vi "Main-e.vi"() -> ()   [LabVIEW 2015]
doc: "This template is for the Queued Message Handler design pattern.\n\nThe Event Handling Loop generates messages based on user interface actions.\n\nThe Message Handling Loop processes messages generated by the Event Handling Loop, or by other messages. The messages are string values, so new messages can be added easily to the Message Cases case structure in the Message Handling Loop. Each message cluster can also provide an optional value for Message Data, which is a variant that can be converted to whatever message-specific data is required."
uses:
  controls/UI Data.ctl
  <vilib>/Platform/TimedLoop/XDataNode/timing_clust.ctl
  <vilib>/Platform/TimedLoop/XDataNode/nitl_modes.ctl
  <vilib>/Platform/TimedLoop/XDataNode/wakeup.ctl
  support/Message Queue/Enqueue Message (Single).vi
  <vilib>/Utility/error.llb/Error Cluster From Error Code.vi
  <vilib>/ErrorRing/Error Ring.xnode
  <vilib>/platform/TimedLoop/XDataNode/XDataNode.xnode
  support/Message Queue/Message Queue.lvlib
  support/User Events/User Events.lvlib
  <userlib>/cameraLibrary/cameraLibrary.lvlib
  <vilib>/Platform/TimedLoop/XDataNode/XDNodeRunTimeDep.lvlib
panel:
  out "status out":u32
  in  "Stop Button":bool
  out "Array Temp":i32
  in  "Set Temp":i32
  out "Image":T1(plugin-control)
  out "loopClosed?":bool
  out "ROIUpdated?":bool
  in  "closeLoopButton":bool
  in  "Subframe":dbl(ring) items=["Slow"=0.01, "Medium"=0.005, "Fast"=0.001]
  in  "Full frame":dbl
  out "Y Fiber Position":i32
  out "X Fiber Pos.":i32
  in  "Y Dimension":i16
  in  "X Dimension":i16
  in  "roiButton":bool
  in  "fullFrameButton":bool
  out "Display":string
  in  "abortButton":bool
  in  "subFrameButton":bool
  in  "Exit":bool
  # "Status indicators"
  # "Loop Closed"
  # "ROI Up-to-date"
  # "Timing parameters"
  # "ROI parameters"
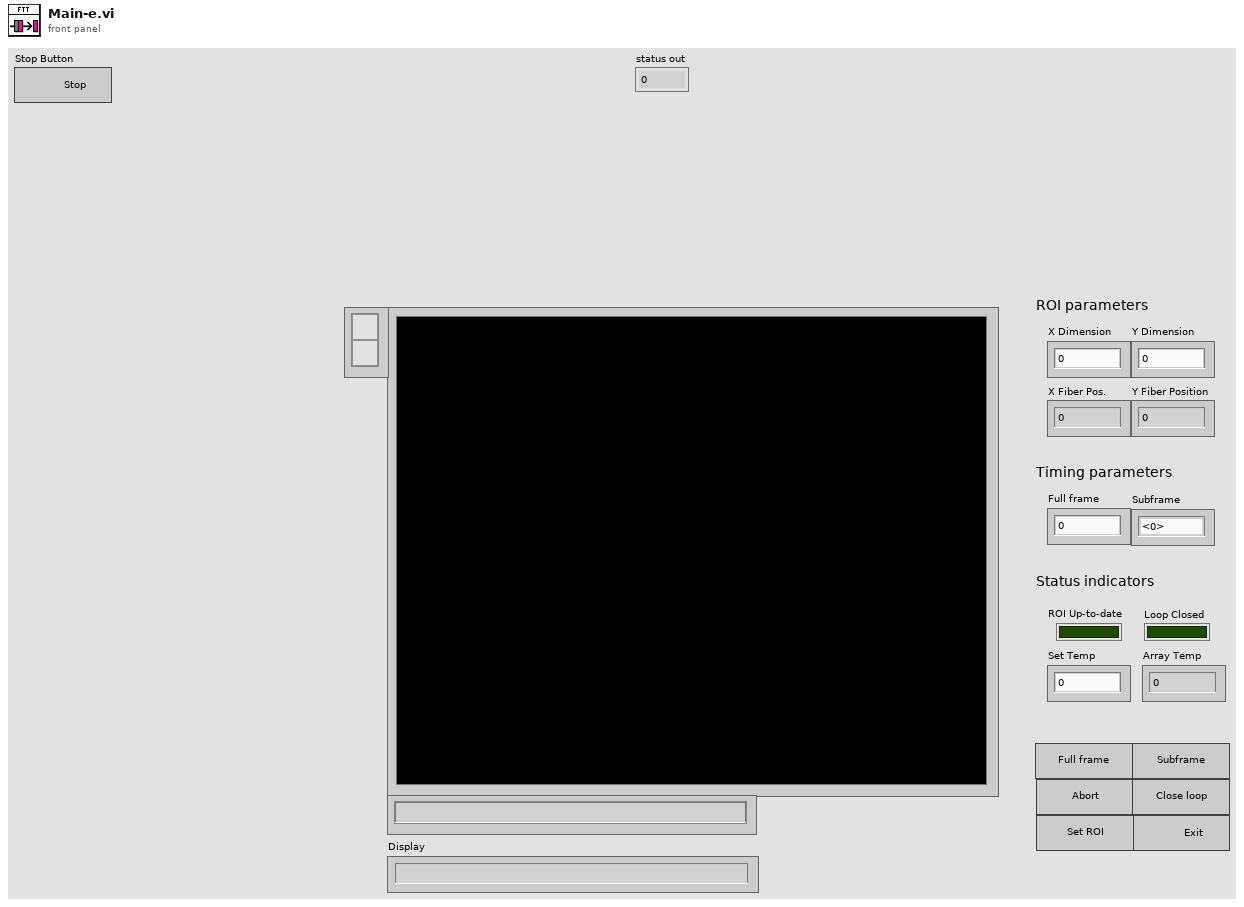
[diagram p1: front panel]
types:
  T1 = typedef "IMAQ Image.ctl" = refnum<image>
  T2 = typedef "Image Type" = u32
  T3 = typedef "UI Data.ctl" = cluster{"full Frame Button Ref":refnum<vi>, "subFrame Button Ref":refnum<vi>, "closed Loop Button Ref":refnum<vi>, "ROI button Ref":refnum<vi>, "abort Button Ref":refnum<vi>, "exit Button Ref":refnum<vi>, "acquiring":bool, " acquiring Ref":refnum<vi>, " ROI Updated Ref":refnum<vi>, "loop Closed Ref":refnum<vi>, "ROI":cluster{"X dimension":i16, "Y dimension":i16, "X binning":i16, "Y binning":i16, "X start":i16, "Y start":i16}, "String <Replace Me>":string, "Data Display Ref":refnum<vi>, "Image Ref":refnum<vi>}
  T4 = typedef "UI Events.ctl" = cluster{"User Event - Stop":refnum<user-event>, "User Event - Abort":refnum<user-event>, "User Event - UpdateTemp":refnum<user-event>}
  T5 = typedef "Message Queue.lvlib/All Message Queues.ctl" = cluster{"UI":refnum<queue>, "DataDisplay":refnum<queue>}
  T6 = typedef "XDNodeRunTimeDep.lvlib/timing_clust.ctl" = cluster{"Expected End [f-1]":u64, "Actual End [f-1]":u64, "Finished Late? [f-1]":bool, "Expected End [i-1]":u64, "Actual End [i-1]":u64, "Finished Late? [i-1]":bool, "Expected Start [i]":u64, "Actual Start [i]":u64, "Expected Start [f]":u64, "Actual Start [f]":u64, "Source Name":string, "Structure Name":string, "Period":i64, "Deadline":i64, "Offset":i64, "Start":i64, "Priority":i32, "Timeout":i32, "Mode":T7, "Wakeup Reason":T8, "Error":errorcluster, "Source Type":string, "Secondary Source Type":string, "Global End Time":u64, "Global Start Time":u64, "Frame Duration":u64, "Iteration Duration":u64, "Assigned CPU":i32, "I/O Scan Engine Mode":u32}
  T7 = typedef "XDNodeRunTimeDep.lvlib/nitl_modes.ctl" = enum32{"No Change", "Process missed periods, maintain original phase", "Discard missed periods, maintain original phase", "Process missed periods, ignore original phase", "Discard missed periods, ignore original phase"}
  T8 = typedef "XDNodeRunTimeDep.lvlib/wakeup.ctl" = enum32{"Normal", "Aborted", "Asynchronous wakeup", "Timing source error", "Timed loop error", "Timeout"}
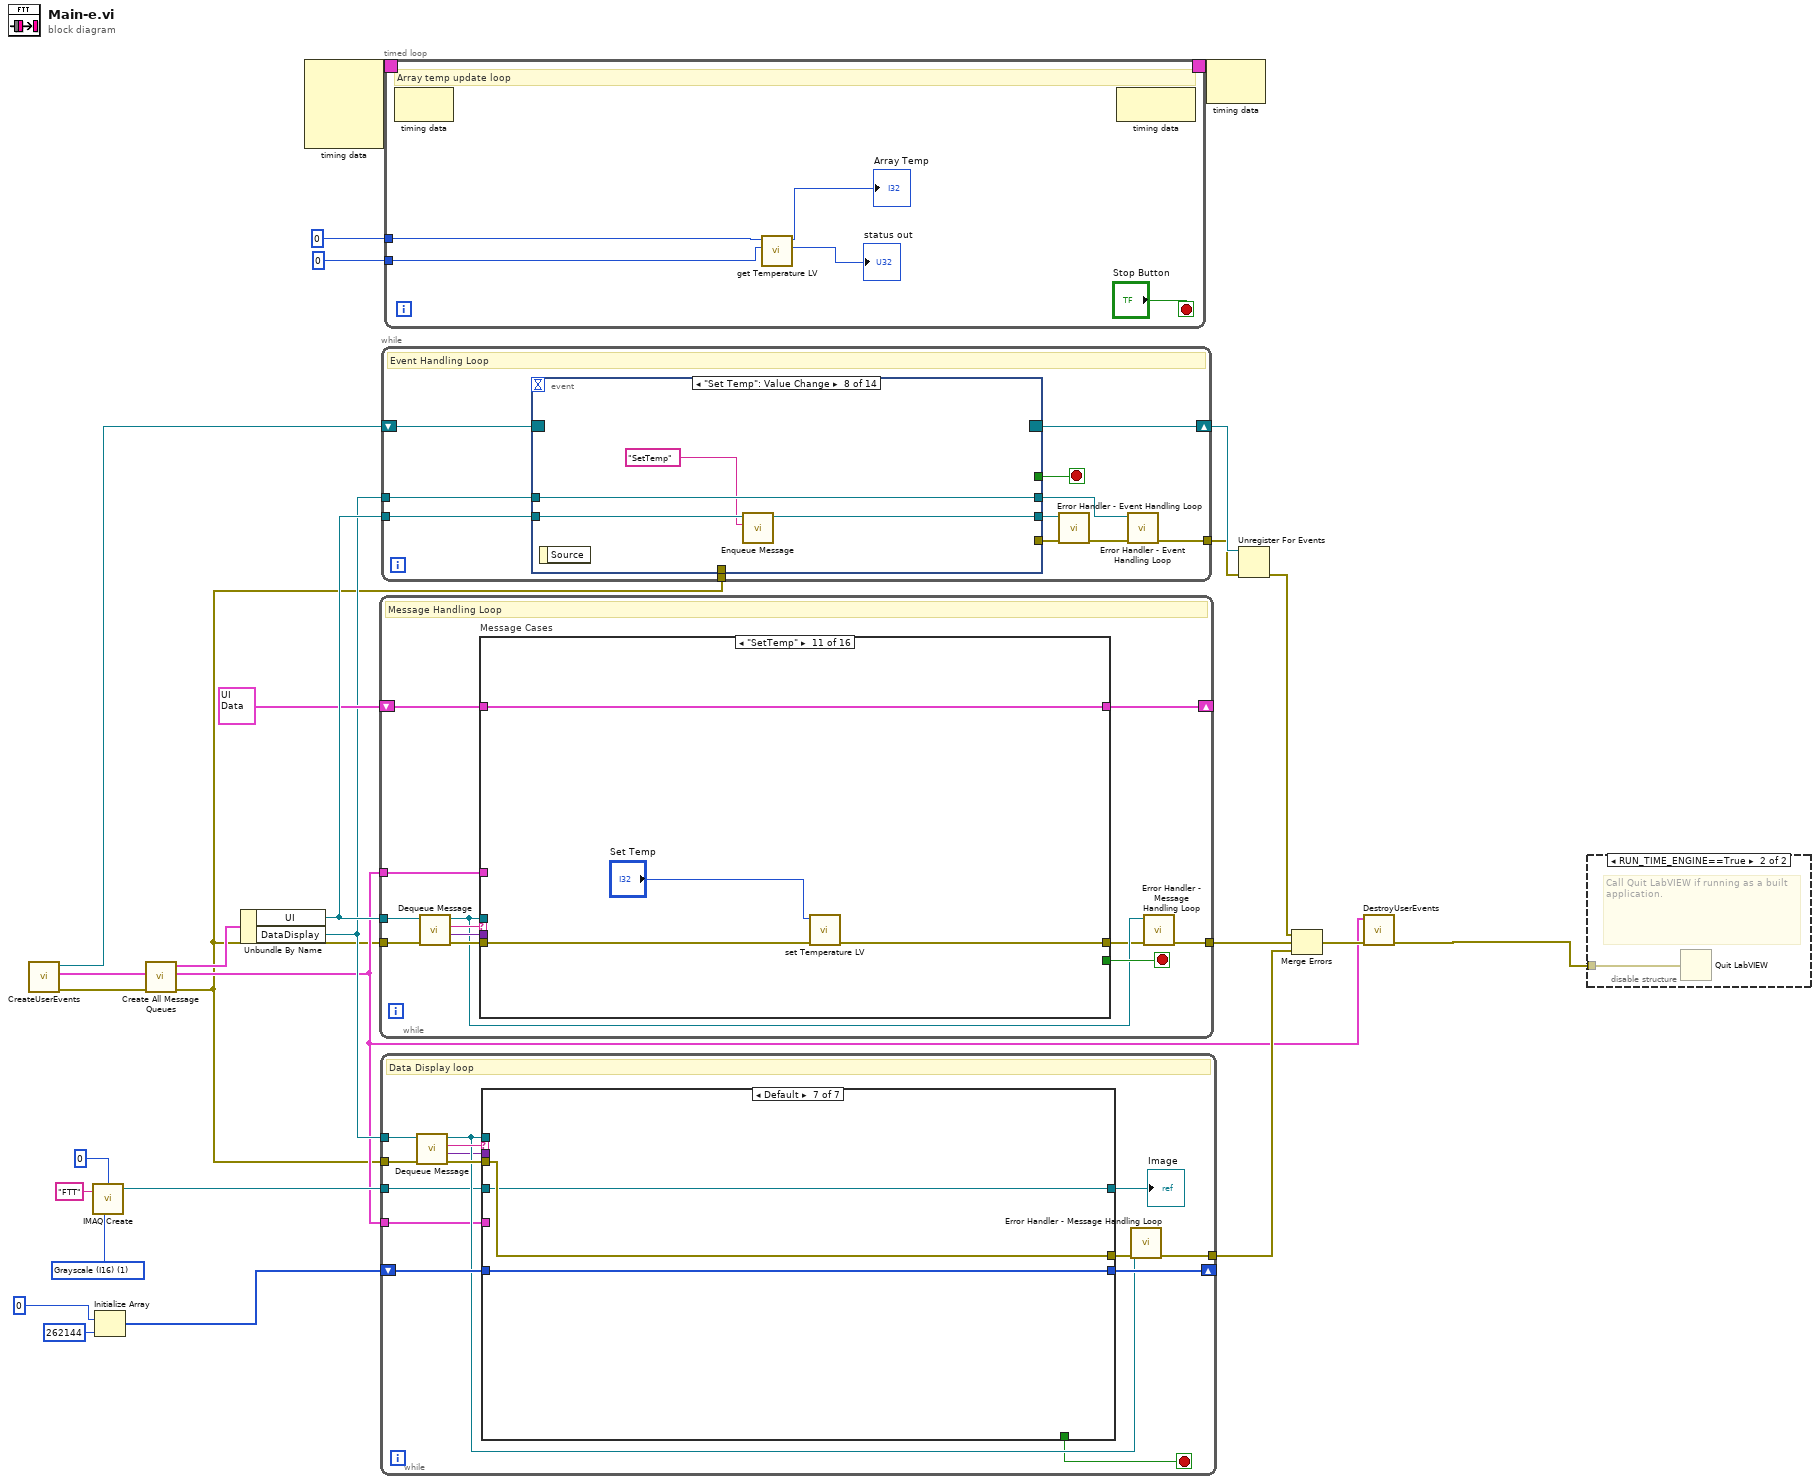
[diagram p0: block diagram]
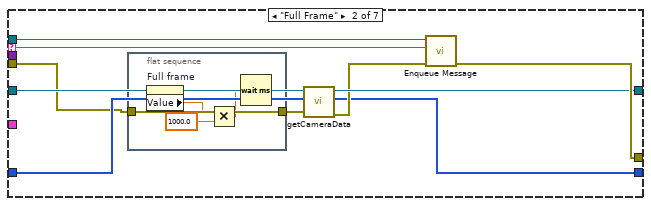
[diagram p3: hidden frame]
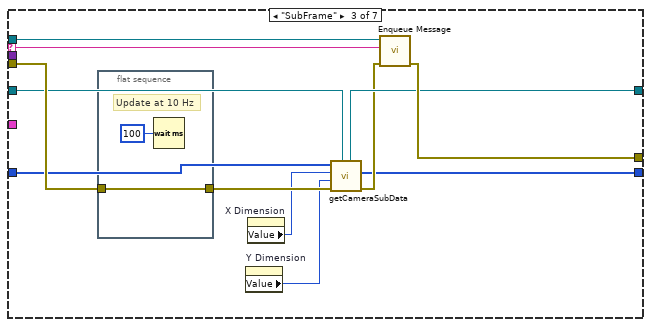
[diagram p4: hidden frame]
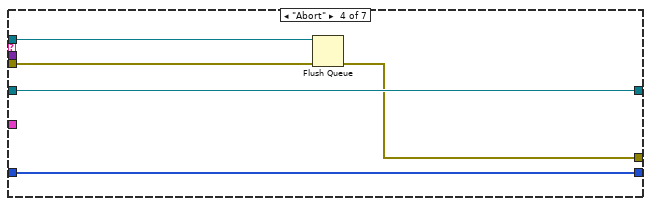
[diagram p5: hidden frame]
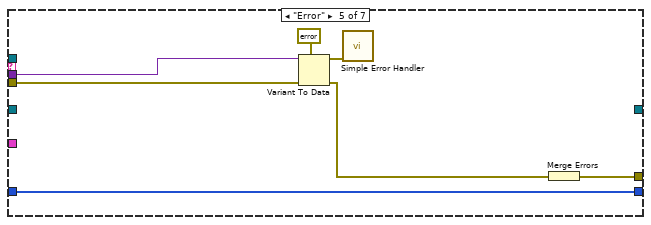
[diagram p6: hidden frame]
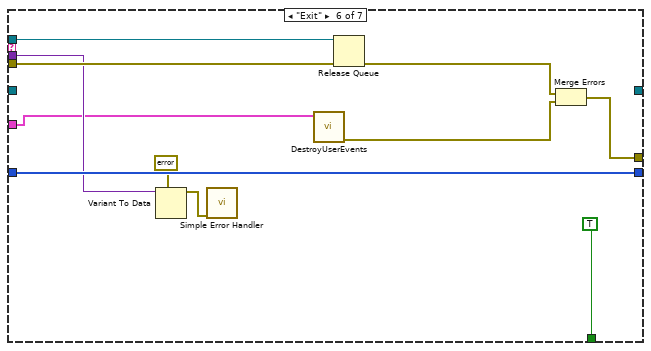
[diagram p7: hidden frame]
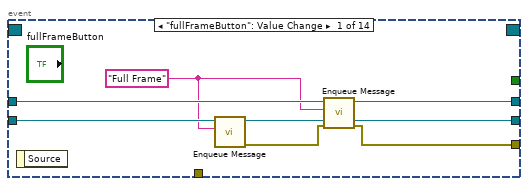
[diagram p9: hidden frame]
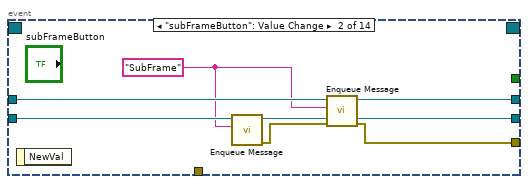
[diagram p10: hidden frame]
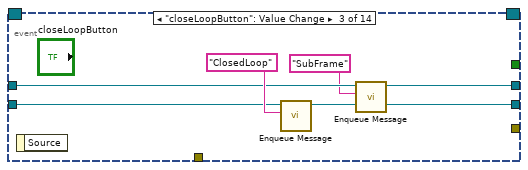
[diagram p11: hidden frame]
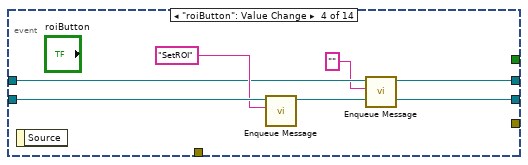
[diagram p12: hidden frame]
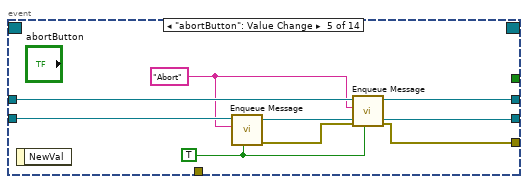
[diagram p13: hidden frame]
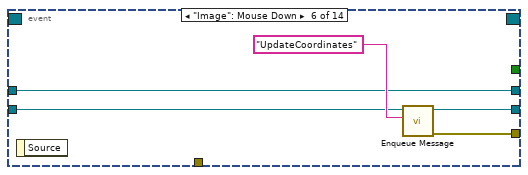
[diagram p14: hidden frame]
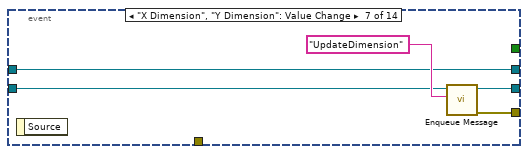
[diagram p15: hidden frame]
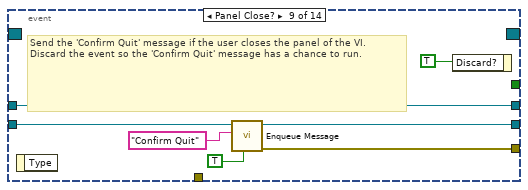
[diagram p16: hidden frame]
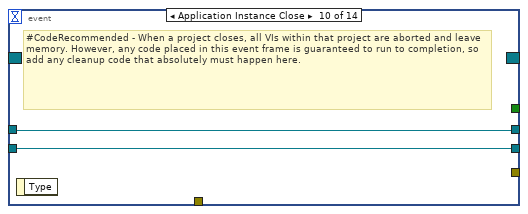
[diagram p17: hidden frame]
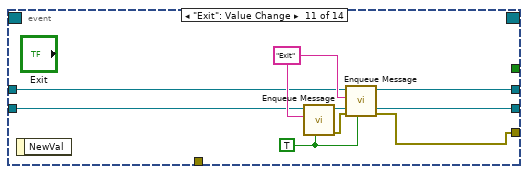
[diagram p18: hidden frame]
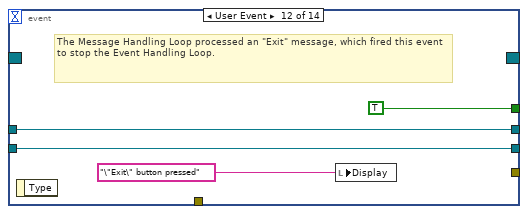
[diagram p19: hidden frame]
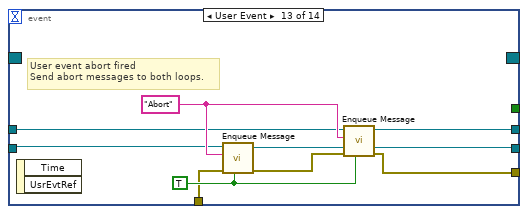
[diagram p20: hidden frame]
diagram:
  w13 = T2 1 items=["Grayscale (U8)", "Grayscale (I16)", "Grayscale (SGL)", "Complex (CSG)", "RGB (U32)", "HSL (U32)", "RGB (U64)", "Grayscale (U16)"] ("Image Type")
  n1 = call "CreateUserEvents.vi"() -> ("error out"=w23:errorcluster, "Event Cluster"=w7:T4, "Event Registration Refnum out"=w19:refnum<event-registration>)  [unwired: 9 in]
  n2 = call "IMAQ Create"("Border Size"=0, "Image Name"="FTT", "Image Type"=w13) -> ("New Image"=w10:T1)  [unwired: 2 in, 1 out]
  n3 = Initialize Array(u32 0, 262144 ("dimension size")) -> (w12:u32[])
  n4 = call "Create All Message Queues.vi"("error in (no error)"=w23) -> ("error out"=w5:errorcluster, "Message Queues out"=w26:T5)  [unwired: 9 in]
  n5 = Unbundle By Name(w26) -> ("UI"=w24:refnum<queue>, "DataDisplay"=w9:refnum<queue>)
  n6 = node-c288() -> (w4:T6)  [unwired: 4 in]
  n7 = while {
    tunnel: w24 -> [w33]
    shift-right: [w28] -> _
    shift-left: T3 {"full Frame Button Ref"=refnum, "subFrame Button Ref"=refnum, "closed Loop Button Ref"=refnum, "ROI button Ref"=refnum, "abort Button Ref"=refnum, "exit Button Ref"=refnum, "acquiring"=FALSE, " acquiring Ref"=refnum, " ROI Updated Ref"=refnum, "loop Closed Ref"=refnum, "ROI"={"X dimension"=0, "Y dimension"=0, "X binning"=0, "Y binning"=0, "X start"=0, "Y start"=0}, "String <Replace Me>"="", "Data Display Ref"=refnum, "Image Ref"=refnum} ("Data Cluster") -> [w38]
    tunnel: [w29] -> w25
    tunnel: w5 -> [w30]
    tunnel: w7 -> [w27]
    stop <- w37 stop-if-true
    # "Message Handling Loop"
    n8 = call "Dequeue Message.vi"("error in (no error)"=w30, "Message Queue"=w33) -> ("error out"=w36:errorcluster, "Message Data"=w34:variant, "Message"=w35:string, "dup Message Queue"=w32:refnum<queue>)  [unwired: 6 in]
    n9 = case "Message Cases" shown="\"SetTemp\"" w35 {
      selector: w35 -> [_ _ w71 _ _ _ _ _ _ _ _ _ _ _ _ w214]
      tunnel: w32 -> [w52 w66 w74 w90 _ _ _ _ _ _ _ _ w190 _ w213 _]
      tunnel: w36 -> [w51 w61 w73 w89 w108 w126 w142 w157 w159 w174 w179 w187 w194 w197 w204 _]
      tunnel: [w55 w67 w72 w93 w107 w125 w142 w157 w163 w175 w178 w181 w192 w195 w209 w215] -> w31
      tunnel: w38 -> [w54 w56 w76 w92 w110 w128 w140 w156 w161 w176 w180 w186 w193 w196 w212 w216]
      tunnel: [w45 w64 w70 w94 w109 w127 w139 w155 w162 w176 w180 w186 w193 w196 w212 w216] -> w28
      tunnel: [_ _ _ _ _ _ _ _ _ _ _ _ _ _ TRUE _] -> w37
      tunnel: w34 -> [_ _ _ _ _ _ _ _ _ w173 _ w185 _ _ w205 _]
      tunnel: w27 -> [_ _ w69 w88 w106 _ _ _ _ _ _ _ _ _ w200 _]
      frame "Initialize" {
        # "Initialize front panel buttons ."
        n10 = control-ref of="fullFrameButton"() -> (w50:refnum<vi>)
        n11 = control-ref of="subFrameButton"() -> (w49:refnum<vi>)
        n12 = control-ref of="closeLoopButton"() -> (w48:refnum<vi>)
        n13 = control-ref of="roiButton"() -> (w47:refnum<vi>)
        n14 = control-ref of="Display"() -> (w39:refnum<vi>)
        n15 = Bundle By Name(cluster=w54, "full Frame Button Ref"=w50, "subFrame Button Ref"=w49, "closed Loop Button Ref"=w48, "ROI button Ref"=w47, "Data Display Ref"=w39) -> (w46:T3)
        n16 = control-ref of="abortButton"() -> (w41:refnum<vi>)
        n17 = control-ref of="Exit"() -> (w42:refnum<vi>)
        n18 = control-ref of="ROIUpdated?"() -> (w40:refnum<vi>)
        n19 = control-ref of="loopClosed?"() -> (w43:refnum<vi>)
        n20 = control-ref of="Image"() -> (w44:refnum<vi>)
        n21 = Bundle By Name(cluster=w46, "abort Button Ref"=w41, "exit Button Ref"=w42, "ROI Updated Ref"=w40, "loop Closed Ref"=w43, "Image Ref"=w44) -> (w45:T3)
        n22 = call-poly "Enqueue Message.vi"("error in (no error)"=w51, "Message"="InitCamera", "Message Queue"=w52) -> ("error out"=w55:errorcluster)  [unwired: 7 in, 1 out]
      }
      frame "InitCamera" {
        w58 = 0.00125 items=["Slow"=0.01, "Medium"=0.035, "Fast"=0.00125] ("Subframe")
        w62 = i16 240 ("ROI.X start")
        w63 = i16 1 ("ROI.X binning")
        w59 = i16 32 ("ROI.X dimension")
        n23 = property on="Subframe" class="Ring (strict)"("Value"=w58) -> ()  [unwired: 2 in, 2 out]
        n24 = Bundle By Name(cluster=w56, "ROI.X dimension"=w59, "ROI.Y dimension"=w59, "ROI.X binning"=w63, "ROI.Y binning"=w63, "ROI.X start"=w62, "ROI.Y start"=w62) -> (w64:T3)
        n25 = call <userlib>:"initialize Camera LV.vi"("error in (no error)"=w61) -> ("error out"=w60:errorcluster)  [unwired: 10 in]
        n26 = property on="Full frame" class="DigNum (strict)"("Value"=0.5 ("Full frame")) -> ()  [unwired: 2 in, 2 out]
        n27 = property on="X Dimension" class="DigNum (strict)"("Value"=w59) -> ()  [unwired: 2 in, 2 out]
        n28 = property on="Y Dimension" class="DigNum (strict)"("Value"=w59) -> ()  [unwired: 2 in, 2 out]
        n29 = call-poly "Enqueue Message.vi"("error in (no error)"=w60, "Message Data"="Camera initialized" ("\"Do Something Else\" button pressed"), "Message"="Update Display", "Message Queue"=w66) -> ("error out"=w67:errorcluster)  [unwired: 6 in, 1 out]
      }
      frame "Full Frame" {
        n30 = Unbundle By Name(w76) -> ("acquiring"=w75:bool)
        n31 = case shown="True" w75 {
          tunnel: w76 -> [w81 w86]
          tunnel: [w81 w87] -> w70
          tunnel: w74 -> [_ _]
          tunnel: w73 -> [w78 w82]
          tunnel: [w77 w83] -> w72
          tunnel: w71 -> [_ _]
          tunnel: w69 -> [w80 _]
          frame True {
            # "Currently acquiring.\nFire user abort event."
            n32 = Unbundle By Name(w80) -> ("User Event - Abort"=w79:refnum<user-event>)
            n33 = call "Fire User Event - Abort.vi"("error in (no error)"=w78, "User Event - Abort"=w79) -> ("error out"=w77:errorcluster)  [unwired: 9 in]
          }
          frame False {
            # "Not currently acquiring.\nStart acquisition\nUpdate display parameters"
            n34 = call <userlib>:"acquire Full Frame LV.vi"("error in (no error)"=w82, "expTime"="Full frame") -> ("error out"=w84:errorcluster)  [unwired: 9 in]
            n35 = call "updateGUIDisplayParams.vi"("error in (no error)"=w84, "Data Cluster in"=w86) -> ("error out"=w83:errorcluster, "Data Cluster out"=w87:T3)  [unwired: 8 in]
          }
        }
      }
      frame "SubFrame" {
        # "Acquire a single frame from the camera"
        n36 = Unbundle By Name(w92) -> ("acquiring"=w91:bool)
        n37 = case shown="False" w91 {
          tunnel: w92 -> [w99 w100]
          tunnel: [w99 w103] -> w94
          tunnel: w90 -> [_ _]
          tunnel: w89 -> [w96 w105]
          tunnel: [w95 w101] -> w93
          tunnel: w88 -> [w98 _]
          frame True {
            # "Currently acquiring.\nFire user abort event.\nAborts current acquisition and stops data display loop"
            n38 = Unbundle By Name(w98) -> ("User Event - Abort"=w97:refnum<user-event>)
            n39 = call "Fire User Event - Abort.vi"("error in (no error)"=w96, "User Event - Abort"=w97) -> ("error out"=w95:errorcluster)  [unwired: 9 in]
          }
          frame False {
            n40 = call <userlib>:"acquire Sub Frame LV.vi"("error in (no error)"=w105, "expTime"="Subframe") -> ("error out"=w102:errorcluster)  [unwired: 9 in]
            n41 = call "updateGUIDisplayParams.vi"("error in (no error)"=w102, "Data Cluster in"=w100) -> ("error out"=w101:errorcluster, "Data Cluster out"=w103:T3)  [unwired: 8 in]
          }
        }
      }
      frame "ClosedLoop" {
        # "Handle closed loop button press. Start process FTT loop."
        n42 = Unbundle By Name(w110) -> ("acquiring"=w111:bool)
        n43 = case shown="True" w111 {
          tunnel: w110 -> [w116 w124]
          tunnel: [w113 w124] -> w109
          tunnel: w108 -> [w119 w121]
          tunnel: [w114 w120] -> w107
          tunnel: w106 -> [_ w123]
          frame False {
            # "Not acquiring, start closed\nloop acquisition"
            n44 = property on="Subframe" class="Ring (strict)"(error in=w119) -> (error out=w118:errorcluster, "Value"=w117:dbl)  [unwired: 1 in, 1 out]
            n45 = call <userlib>:"acquire Closed Loop LV.vi"("error in (no error)"=w118, "expTime"=w117) -> ("error out"=w115:errorcluster)  [unwired: 9 in]
            n46 = call "updateGUIDisplayParams.vi"("error in (no error)"=w115, "Data Cluster in"=w116) -> ("error out"=w114:errorcluster, "Data Cluster out"=w113:T3)  [unwired: 8 in]
            "loopClosed?" <- TRUE ("loopClosed?")
          }
          frame True {
            # "Currently acquiring.\nFire user abort event.\nAborts current acquisition and stops data display loop"
            n47 = Unbundle By Name(w123) -> ("User Event - Abort"=w122:refnum<user-event>)
            n48 = call "Fire User Event - Abort.vi"("error in (no error)"=w121, "User Event - Abort"=w122) -> ("error out"=w120:errorcluster)  [unwired: 9 in]
          }
        }
      }
      frame "SetROI" {
        # "Program camera with ROI values."
        n49 = Unbundle By Name(w128) -> ("acquiring"=w129:bool)
        n50 = case shown="True" w129 {
          tunnel: w128 -> [w131 w136]
          tunnel: [w131 w135] -> w127
          tunnel: w126 -> [w130 w134]
          tunnel: [w130 w133] -> w125
          frame True {
            # "Acquiring, do nothing\nShould be fixed with button masking"
          }
          frame False {
            # "Not acquiring, set ROI"
            n51 = call "setROI.vi"("error in (no error)"=w134, "FTTclusterIn"=w136) -> ("error out"=w133:errorcluster, "FTTclusterOut"=w135:T3)  [unwired: 8 in]
            "ROIUpdated?" <- TRUE ("ROIUpdated?")
          }
        }
      }
      frame "UpdateCoordinates" {
        # "Image clicked. If Acquiring, update coordinates.\nSignal ROI updated is false"
        n52 = Unbundle By Name(w140) -> ("Image Ref"=w137:refnum<vi>, "acquiring"=w141:bool, "ROI Updated Ref"=w138:refnum<vi>)
        n53 = case shown="True" w141 {
          tunnel: w140 -> [w143 w151]
          tunnel: [w143 w150] -> w139
          tunnel: w138 -> [_ w146]
          tunnel: w137 -> [_ w144]
          frame False {
          }
          frame True {
            n54 = property class="ImageControl"(reference=w144) -> ("Last Mouse Position"=w152:cluster{"X":i32, "Y":i32})  [unwired: 1 in, 2 out]
            n55 = property class="Bool (strict)"(reference=w146, "Value"=FALSE) -> ()  [unwired: 1 in, 2 out]
            n56 = call "checkROIStart.vi"("lastClickPosition"=w152, "FTTDataClusterIn"=w151) -> ("coords"=w149:cluster{"X":i32, "Y":i32}, "FTTDataClusterOut"=w150:T3)  [unwired: 8 in]
            n57 = Unbundle By Name(w149) -> ("X"=→"X Fiber Pos.":i32, "Y"=→"Y Fiber Position":i32)
          }
        }
      }
      frame "UpdateDimension" {
        n58 = Bundle By Name(cluster=w156, "ROI.X dimension"="X Dimension", "ROI.Y dimension"="Y Dimension") -> (w155:T3)
      }
      frame "Abort" {
        # "Abort camera acquistion and update GUI."
        n59 = Unbundle By Name(w161) -> ("acquiring"=w160:bool)
        n60 = call <userlib>:"abort Acquisition LV.vi"("error in (no error)"=w159) -> ("error out"=w158:errorcluster)  [unwired: 10 in]
        n61 = case shown="True" w160 {
          tunnel: w158 -> [w165 w169]
          tunnel: [w165 w168] -> w163
          tunnel: [w164 w166] -> w162
          tunnel: w161 -> [w164 w167]
          frame False {
          }
          frame True {
            n62 = call "updateGUIDisplayParams.vi"("error in (no error)"=w169, "Data Cluster in"=w167) -> ("error out"=w168:errorcluster, "Data Cluster out"=w166:T3)  [unwired: 8 in]
          }
        }
      }
      frame "Update Display" {
        # "Update Display - Convert the message data to a string to display in the Data Display indicator."
        n63 = Variant To Data(error in=w174, type="", Variant=w173) -> (data=→"Display":string, error out=w171:errorcluster)
        n64 = Merge Errors(w171) -> (w175:errorcluster)
      }
      frame "SetTemp" {
        n65 = call <userlib>:"set Temperature LV.vi"("error in (no error)"=w179, "setTemp"="Set Temp") -> ("error out"=w178:errorcluster)  [unwired: 9 in]
      }
      frame "Error" {
        # "#CodeRecommended - If you ever change the name of this \"Error\" message, you'll need to update the name in the Check Loop Error.vi as well."
        # "#CodeRecommended - Consider creating a system for logging errors in some way. These errors are for notification purposes only. Handling of specific errors should be performed in the message frames that generated the error."
        # "Error - Display an error dialog. This message is sent by the \"Error Handler\" VIs at the end of other loops in this application."
        n66 = Variant To Data(error in=w187, type=errorcluster {"status"=FALSE, "code"=0, "source"=""} ("error constant"), Variant=w185) -> (data=w183:errorcluster, error out=w182:errorcluster)
        n67 = call <vilib>:"Simple Error Handler.vi"("error in (no error)"=w183) -> ()  [unwired: 4 in, 5 out]
        n68 = Merge Errors(w182) -> (w181:errorcluster)
      }
      frame "Confirm Quit" {
        # "#CodeNeeded - If you want to provide an \"Are you sure\" dialog (or some other notification) before the application exits, place that code here. This message is typically sent from a Panel Close? event."
        # "Confirm Quit - Message that can confirm whether or not the user wants to exit the application."
        n69 = call-poly "Enqueue Message.vi"("Priority Message? (F)"=TRUE, "error in (no error)"=w194, "Message"="Exit", "Message Queue"=w190) -> ("error out"=w191:errorcluster)  [unwired: 6 in, 1 out]
        n70 = Merge Errors(w191) -> (w192:errorcluster)
      }
      frame "---Copy This Frame---" {
        # "Duplicate this frame when creating new messages.  Change this comment in the duplicated frame to describe this message."
        n71 = Merge Errors(w197) -> (w195:errorcluster)
      }
      frame "Exit" {
        # "Stop the VI"
        # "#CodeNeeded - Add any required cleanup code here. Note that if 'Exit' was called as a result of an error, an error dialog will be displayed. Add any custom error handling for an 'Exit' condition here as well."
        # "Exit - Exit the application."
        n72 = Unbundle By Name(w200) -> ("User Event - Stop"=w199:refnum<user-event>, "User Event - Abort"=w198:refnum<user-event>)
        n73 = Variant To Data(type=errorcluster {"status"=FALSE, "code"=0, "source"=""} ("error constant"), Variant=w205) -> (data=w206:errorcluster)  [unwired: 1 in, 1 out]
        n74 = call <vilib>:"Simple Error Handler.vi"("error in (no error)"=w206) -> ()  [unwired: 4 in, 5 out]
        n75 = call <userlib>:"abort Acquisition LV.vi"("error in (no error)"=w204) -> ("error out"=w203:errorcluster)  [unwired: 10 in]
        n76 = call <userlib>:"shutdown Camera LV.vi"("error in (no error)"=w203) -> ("error out"=w202:errorcluster)  [unwired: 10 in]
        n77 = call "Destroy User Event -Abort.vi"("User Event - Abort"=w198) -> ("error out"=w201:errorcluster)  [unwired: 10 in]
        n78 = call "Fire User Event - Stop.vi"("error in (no error)"=w201, "User Event - Stop"=w199) -> ("error out"=w208:errorcluster)  [unwired: 9 in]
        n79 = Release Queue(queue=w213, error in (no error)=w202) -> (error out=w210:errorcluster)  [unwired: 1 in, 2 out]
        n80 = Merge Errors(w208, w210) -> (w209:errorcluster)
      }
      frame Default {
        # "'Default' case only runs if there is a message that isn't defined in any of the other cases.  Output a programming error."
        n81 = xnode "Error Ring"("parameter 0"=w214) -> ("error out"=w215:errorcluster)
      }
    }
    n82 = call "Error Handler - Message Handling Loop.vi"("error in (no error)"=w31, "Message Queue"=w32) -> ("dup error in"=w29:errorcluster)  [unwired: 8 in, 1 out]
  }
  n83 = while {
    tunnel: w9 -> [w236]
    tunnel: w5 -> [w235]
    tunnel: [w233] -> w11
    shift-right: [w230] -> _
    shift-left: w12 -> [w237]
    tunnel: w10 -> [w227]
    tunnel: w7 -> [w224]
    stop <- w228 stop-if-true
    # "Data Display loop"
    n84 = call "Dequeue Message.vi"("error in (no error)"=w235, "Message Queue"=w236) -> ("error out"=w231:errorcluster, "Message Data"=w226:variant, "Message"=w234:string, "dup Message Queue"=w229:refnum<queue>)  [unwired: 6 in]
    n85 = case shown="Default" w234 {
      selector: w234 -> [_ w249 w265 _ _ _ _]
      tunnel: w237 -> [w240 w244 w261 w271 w276 w286 w293]
      tunnel: w229 -> [_ w250 w266 w273 _ w291 _]
      tunnel: [w239 w248 w264 w269 w274 w289 w294] -> w232
      tunnel: w231 -> [w239 w242 w263 w272 w278 w290 w294]
      tunnel: [w238 w246 w259 w270 _ _ w292] -> w225
      tunnel: [w240 w243 w257 w271 w276 w286 w293] -> w230
      tunnel: [_ _ _ _ _ TRUE _] -> w228
      tunnel: w227 -> [w238 w247 w260 w270 _ _ w292]
      tunnel: w226 -> [_ _ _ _ w277 w284 _]
      tunnel: w224 -> [_ _ _ _ _ w281 _]
      frame "Initialize" {
      }
      frame "Full Frame" {
        n86 = flat-sequence {
          tunnel: w242 -> [w254]
          tunnel: [w254] -> w241
          frame #0 {
            n87 = property on="Full frame" class="DigNum (strict)"() -> ("Value"=w252:dbl)  [unwired: 2 in, 2 out]
            n88 = Multiply(x=w252, y=1000.0) -> (x*y=w253:dbl)
            n89 = Wait (ms)(milliseconds to wait=w253) -> ()  [unwired: 1 out]
          }
        }
        n90 = call "getCameraData.vi"("error in (no error)"=w241, "Array"=w244, "Refnum in"=w247) -> ("error out"=w245:errorcluster, "arrayOut"=w243:u32[], "Refnum out"=w246:T1)  [unwired: 6 in]
        n91 = call-poly "Enqueue Message.vi"("error in (no error)"=w245, "Message"=w249, "Message Queue"=w250) -> ("error out"=w248:errorcluster)  [unwired: 7 in, 1 out]
      }
      frame "SubFrame" {
        n92 = flat-sequence {
          tunnel: w263 -> [w267]
          tunnel: [w267] -> w262
          frame #0 {
            # "Update at 10 Hz"
            n93 = Wait (ms)(milliseconds to wait=u32 100) -> ()  [unwired: 1 out]
          }
        }
        n94 = property on="Y Dimension" class="DigNum (strict)"() -> ("Value"=w256:i16)  [unwired: 2 in, 2 out]
        n95 = property on="X Dimension" class="DigNum (strict)"() -> ("Value"=w255:i16)  [unwired: 2 in, 2 out]
        n96 = call "getCameraSubData.vi"("Refnum in"=w260, "error in (no error)"=w262, "VDim"=w256, "HDim"=w255, "arrayIn"=w261) -> ("error out"=w258:errorcluster, "arrayOut"=w257:u32[], "Refnum out"=w259:T1)  [unwired: 4 in]
        n97 = call-poly "Enqueue Message.vi"("error in (no error)"=w258, "Message"=w265, "Message Queue"=w266) -> ("error out"=w264:errorcluster)  [unwired: 7 in, 1 out]
      }
      frame "Abort" {
        n98 = Flush Queue(queue=w273, error in (no error)=w272) -> (error out=w269:errorcluster)  [unwired: 2 out]
      }
      frame "Error" {
        n99 = Variant To Data(error in=w278, type=errorcluster {"status"=FALSE, "code"=0, "source"=""} ("error constant"), Variant=w277) -> (data=w279:errorcluster, error out=w275:errorcluster)
        n100 = call <vilib>:"Simple Error Handler.vi"("error in (no error)"=w279) -> ()  [unwired: 4 in, 5 out]
        n101 = Merge Errors(w275) -> (w274:errorcluster)
      }
      frame "Exit" {
        n102 = Variant To Data(type=errorcluster {"status"=FALSE, "code"=0, "source"=""} ("error constant"), Variant=w284) -> (data=w285:errorcluster)  [unwired: 1 in, 1 out]
        n103 = call <vilib>:"Simple Error Handler.vi"("error in (no error)"=w285) -> ()  [unwired: 4 in, 5 out]
        n104 = call "DestroyUserEvents.vi"("Event Cluster"=w281) -> ("error out"=w288:errorcluster)  [unwired: 10 in]
        n105 = Release Queue(queue=w291, error in (no error)=w290) -> (error out=w282:errorcluster)  [unwired: 1 in, 2 out]
        n106 = Merge Errors(w282, w288) -> (w289:errorcluster)
      }
      frame Default {
      }
    }
    "Image" <- w225
    n107 = call "Error Handler - Message Handling Loop.vi"("error in (no error)"=w232, "Message Queue"=w229) -> ("dup error in"=w233:errorcluster)  [unwired: 8 in, 1 out]
  }
  n108 = while {
    tunnel: w24 -> [w305]
    shift-right: [w303] -> w22
    shift-left: w19 -> [w304]
    tunnel: [w298] -> w20
    tunnel: w9 -> [w300]
    tunnel: w5 -> [w295]
    stop <- w302 stop-if-true
    # "Event Handling Loop"
    n109 = event shown="[7] \"Set Temp\": Value Change" {
      selector: w304 -> [_ _ _ _ _ _ _ _ _ _ _ _ _ _]
      dyn-events: [_ _ _ _ _ _ _ _ _ _ _ _ _ _] -> w303
      timeout: _ -> [_ _ _ _ _ _ _ _ _ _ _ _ _ _]
      tunnel: [_ _ _ _ _ _ _ _ _ _ _ TRUE ("Discard?") _ _] -> w302
      tunnel: w305 -> [w312 w319 w324 w331 w339 w343 w348 w352 w359 w362 w366 w374 w378 w385]
      tunnel: [w308 w315 _ _ w334 w341 w346 _ w358 _ w363 _ w376 _] -> w296
      tunnel: [w311 w318 w323 w330 w338 w342 w347 w351 w357 w362 w370 w374 w379 w385] -> w301
      tunnel: w300 -> [w310 w317 w321 w328 w337 w340 w345 w353 w354 w361 w365 w371 w377 w384]
      tunnel: [w307 w313 w322 w327 w335 w340 w345 w353 w354 w361 w367 w371 w380 w384] -> w297
      tunnel: w295 -> [_ _ _ _ _ _ _ _ _ _ _ _ w375 _]
      event "fullFrameButton": Value Change {
        w306 = "Full Frame" ("Message")
        n110 = event-data() -> ()  [unwired: 1 in, 1 out]
        n111 = call-poly "Enqueue Message.vi"("Message"=w306, "Message Queue"=w312) -> ("error out"=w309:errorcluster, "dup Message Queue"=w311:refnum<queue>)  [unwired: 8 in]
        n112 = call-poly "Enqueue Message.vi"("error in (no error)"=w309, "Message"=w306, "Message Queue"=w310) -> ("error out"=w308:errorcluster, "dup Message Queue"=w307:refnum<queue>)  [unwired: 7 in]
      }
      event "subFrameButton": Value Change {
        w314 = "SubFrame" ("Message")
        n113 = event-data() -> ()  [unwired: 1 in, 1 out]
        n114 = call-poly "Enqueue Message.vi"("Message"=w314, "Message Queue"=w319) -> ("error out"=w316:errorcluster, "dup Message Queue"=w318:refnum<queue>)  [unwired: 8 in]
        n115 = call-poly "Enqueue Message.vi"("error in (no error)"=w316, "Message"=w314, "Message Queue"=w317) -> ("error out"=w315:errorcluster, "dup Message Queue"=w313:refnum<queue>)  [unwired: 7 in]
      }
      event "closeLoopButton": Value Change {
        n116 = event-data() -> ()  [unwired: 1 in, 1 out]
        n117 = call-poly "Enqueue Message.vi"("Message"="ClosedLoop", "Message Queue"=w324) -> ("dup Message Queue"=w323:refnum<queue>)  [unwired: 8 in, 1 out]
        n118 = call-poly "Enqueue Message.vi"("Message"="SubFrame", "Message Queue"=w321) -> ("dup Message Queue"=w322:refnum<queue>)  [unwired: 8 in, 1 out]
      }
      event "roiButton": Value Change {
        n119 = event-data() -> ()  [unwired: 1 in, 1 out]
        n120 = call-poly "Enqueue Message.vi"("Message"="SetROI", "Message Queue"=w331) -> ("dup Message Queue"=w330:refnum<queue>)  [unwired: 8 in, 1 out]
        n121 = call-poly "Enqueue Message.vi"("Message"="", "Message Queue"=w328) -> ("dup Message Queue"=w327:refnum<queue>)  [unwired: 8 in, 1 out]
      }
      event "abortButton": Value Change {
        w332 = TRUE ("Priority Message? (F)")
        w333 = "Abort" ("Message")
        n122 = event-data() -> ()  [unwired: 1 in, 1 out]
        n123 = call-poly "Enqueue Message.vi"("Priority Message? (F)"=w332, "Message"=w333, "Message Queue"=w339) -> ("error out"=w336:errorcluster, "dup Message Queue"=w338:refnum<queue>)  [unwired: 7 in]
        n124 = call-poly "Enqueue Message.vi"("Priority Message? (F)"=w332, "error in (no error)"=w336, "Message"=w333, "Message Queue"=w337) -> ("error out"=w334:errorcluster, "dup Message Queue"=w335:refnum<queue>)  [unwired: 6 in]
      }
      event "Image": Mouse Down {
        n125 = event-data() -> ()  [unwired: 1 in, 1 out]
        n126 = call-poly "Enqueue Message.vi"("Message"="UpdateCoordinates", "Message Queue"=w343) -> ("error out"=w341:errorcluster, "dup Message Queue"=w342:refnum<queue>)  [unwired: 8 in]
      }
      event "X Dimension", "Y Dimension": Value Change {
        n127 = event-data() -> ()  [unwired: 1 in, 1 out]
        n128 = call-poly "Enqueue Message.vi"("Message"="UpdateDimension", "Message Queue"=w348) -> ("error out"=w346:errorcluster, "dup Message Queue"=w347:refnum<queue>)  [unwired: 8 in]
      }
      event "Set Temp": Value Change {
        n129 = event-data() -> ()  [unwired: 1 in, 1 out]
        n130 = call-poly "Enqueue Message.vi"("Message"="SetTemp", "Message Queue"=w352) -> ("dup Message Queue"=w351:refnum<queue>)  [unwired: 8 in, 1 out]
      }
      event Panel Close? {
        # "Send the 'Confirm Quit' message if the user closes the panel of the VI. Discard the event so the 'Confirm Quit' message has a chance to run."
        n131 = event-data() -> ()  [unwired: 1 in, 1 out]
        n132 = call-poly "Enqueue Message.vi"("Priority Message? (F)"=TRUE, "Message"="Confirm Quit", "Message Queue"=w359) -> ("error out"=w358:errorcluster, "dup Message Queue"=w357:refnum<queue>)  [unwired: 7 in]
        n133 = event-data("Discard?"=TRUE) -> ()  [unwired: 1 in, 1 out]
      }
      event Application Instance Close {
        # "#CodeRecommended - When a project closes, all VIs within that project are aborted and leave memory. However, any code placed in this event frame is guaranteed to run to completion, so add any cleanup code that absolutely must happen here."
        n134 = event-data() -> ()  [unwired: 1 in, 1 out]
      }
      event "Exit": Value Change {
        w364 = TRUE ("Priority Message? (F)")
        w368 = "Exit" ("Message")
        n135 = event-data() -> ()  [unwired: 1 in, 1 out]
        n136 = call-poly "Enqueue Message.vi"("Priority Message? (F)"=w364, "Message"=w368, "Message Queue"=w366) -> ("error out"=w369:errorcluster, "dup Message Queue"=w370:refnum<queue>)  [unwired: 7 in]
        n137 = call-poly "Enqueue Message.vi"("Priority Message? (F)"=w364, "error in (no error)"=w369, "Message"=w368, "Message Queue"=w365) -> ("error out"=w363:errorcluster, "dup Message Queue"=w367:refnum<queue>)  [unwired: 6 in]
      }
      event User Event {
        # "The Message Handling Loop processed an \"Exit\" message, which fired this event to stop the Event Handling Loop."
        n138 = event-data() -> ()  [unwired: 1 in, 1 out]
        n139 = local write "Display"("\"Exit\" button pressed" ("VI Stopped")) -> ()
      }
      event User Event {
        w381 = TRUE ("Priority Message? (F)")
        w382 = "Abort" ("Message")
        # "User event abort fired\nSend abort messages to both loops."
        n140 = event-data() -> ()  [unwired: 1 in, 2 out]
        n141 = call-poly "Enqueue Message.vi"("Priority Message? (F)"=w381, "error in (no error)"=w375, "Message"=w382, "Message Queue"=w378) -> ("error out"=w383:errorcluster, "dup Message Queue"=w379:refnum<queue>)  [unwired: 6 in]
        n142 = call-poly "Enqueue Message.vi"("Priority Message? (F)"=w381, "error in (no error)"=w383, "Message"=w382, "Message Queue"=w377) -> ("error out"=w376:errorcluster, "dup Message Queue"=w380:refnum<queue>)  [unwired: 6 in]
      }
      event User Event {
        n143 = event-data() -> ()  [unwired: 1 in, 1 out]
      }
    }
    n144 = call "Error Handler - Event Handling Loop.vi"("error in (no error)"=w296, "Message Queue"=w301) -> ("dup error in"=w299:errorcluster)  [unwired: 8 in, 1 out]
    n145 = call "Error Handler - Event Handling Loop.vi"("error in (no error)"=w299, "Message Queue"=w297) -> ("dup error in"=w298:errorcluster)  [unwired: 8 in, 1 out]
  }
  n146 = timed-loop "Timed Loop" {
    timing: w4 -> [_]
    timing-out: [_] -> w3
    tunnel: 0 ("temperature") -> [w388]
    tunnel: u32 0 ("status") -> [w387]
    stop <- "Stop Button" stop-if-true
    # "Array temp update loop"
    n147 = node-c288() -> ()  [unwired: 1 in, 1 out]
    n148 = call <userlib>:"get Temperature LV.vi"("status"=w387, "temperature"=w388) -> ("status out"=→"status out":u32, "temperature out"=→"Array Temp":i32)  [unwired: 7 in, 1 out]
    n149 = node-c288() -> ()  [unwired: 1 in, 1 out]
  }
  n150 = node-c288(w3) -> ()  [unwired: 1 out]
  n151 = Unregister For Events(event registration refnum=w22, error in=w20) -> (error out=w18:errorcluster)
  n152 = Merge Errors(w18, w25, w11) -> (w8:errorcluster)
  n153 = call "DestroyUserEvents.vi"("error in (no error)"=w8, "Event Cluster"=w7) -> ("error out"=w6:errorcluster)  [unwired: 9 in]
  n154 = disable-structure shown="RUN_TIME_ENGINE==True" {
    disable-tunnel: w6 -> [_ w393]
    frame condition #0 (active) {
    }
    frame condition #1 {
      # "Call Quit LabVIEW if running as a built application."
      n155 = Quit LabVIEW(quit? (T)=w393) -> ()
    }
  }
